vi "Translation3d_Create_DistAng.vi"(10 "Angle_Rotation3d":T1={"Q_quaternion"={"R"=1.0, "V"=[0.0, 0.0, 0.0]}}, 11 "Distance":dbl) -> (3 "TRANSLATION3D":T3 {"Z" format="%14.3f"; "Y" format="%14.3f"; "X" format="%14.3f"})   [LabVIEW 2019, in "Trajectory_Library.lvlib"]
doc: "Constructs a Translation3d with the provided distance and angle. This is essentially converting from polar coordinates to Cartesian coordinates.\n\nParameters:\n - Dist - Distance.\n - Ang - Rotation3d representing the angle.\n\nReturns\n - TRANSLATION3d - The TRANSLATION3d data structure"
uses:
  Trajectory_Library.lvlib
  TypeDef/QUATERNION.ctl
  TypeDef/ROTATION3D.ctl
  TypeDef/TRANSLATION3D.ctl
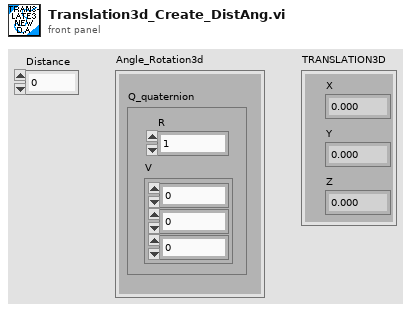
[diagram p1: front panel]
types:
  T1 = typedef "Trajectory_Library.lvlib/ROTATION3D.ctl" = cluster{"Q_quaternion":T2}
  T2 = typedef "Trajectory_Library.lvlib/QUATERNION.ctl" = cluster{"R":dbl, "V":dbl[]}
  T3 = typedef "Trajectory_Library.lvlib/TRANSLATION3D.ctl" = cluster{"X":dbl, "Y":dbl, "Z":dbl}
  T4 = typedef "WPILib_Math.lvlib/TRANSLATION3D.ctl" = cluster{"X":dbl, "Y":dbl, "Z":dbl}
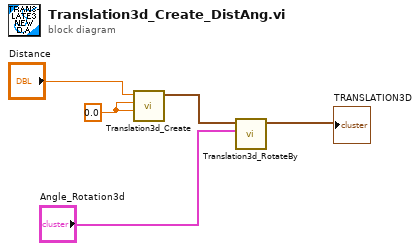
[diagram p0: block diagram]
diagram:
  w4 = 0.0 ("Y")
  n1 = call "Translation3d_Create.vi"("Z"=w4, "Y"=w4, "X"="Distance") -> ("TRANSLATION3D"=w3:T4)  [unwired: 8 in]
  n2 = call "Translation3d_RotateBy.vi"("other Rot3d"="Angle_Rotation3d", "in Translation3D"=w3) -> ("out Translation3d"=→"TRANSLATION3D":T3)  [unwired: 9 in]
